vi "GSP_Monitor_handler.vi"(4 "Mode":u16(ring) items=["External", "Internal"], 5 "error in (no error)":errorcluster, 6 "Action":T1, 7 "Motor#":u8, 8 "Monitor Name":string) -> (0 "error out":errorcluster, 2 "Motor# dup":u8)   [LabVIEW 2015]
doc: "Provides an interface for launching and shutting down Silvermax motor monitors. See the action descriptions below:\n\nLaunch - Supply inputs for monitor name (something descriptive), motor#, and mode (encoder type)\n\nShutdown - Shutdown the motor monitor supplied by Motor#\n\nShutdown All - Shutdown all running motor monitors\n\nShow - Open the front panel of the motor monitor supplied by Motor#\n\nHide - Close the front panel of the motor monitor supplied by Motor#"
uses:
  handler_actions.ctl
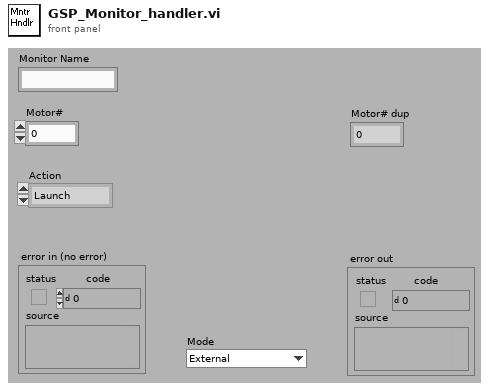
[diagram p1: front panel]
types:
  T1 = typedef "handler_actions.ctl" = enum16{"Launch", "Shutdown All", "Shutdown"}
  T2 = cluster{"Control Name":string, "type string":i16[], "data string":string}
  T3 = cluster{string, "type string":i16[], "data string":string}
  T4 = cluster{"Control Name":string, "type string":i16[], "data string":string}[]
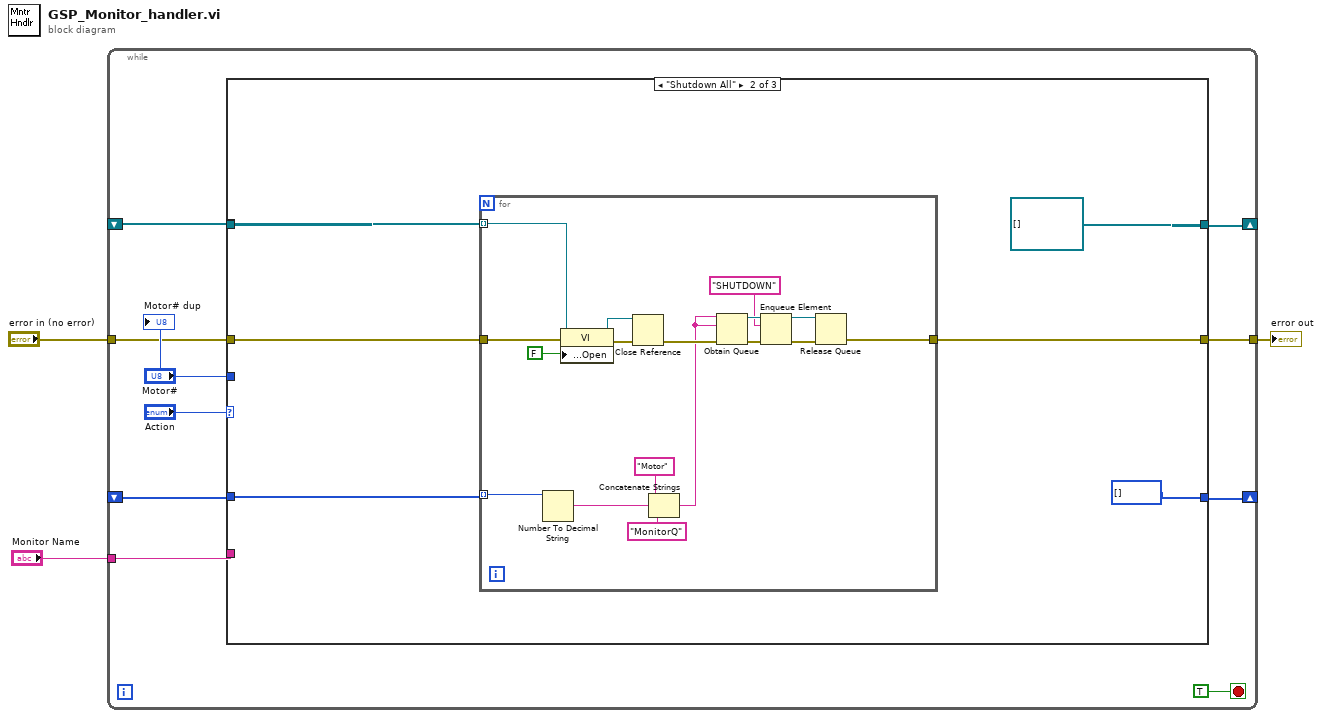
[diagram p0: block diagram]
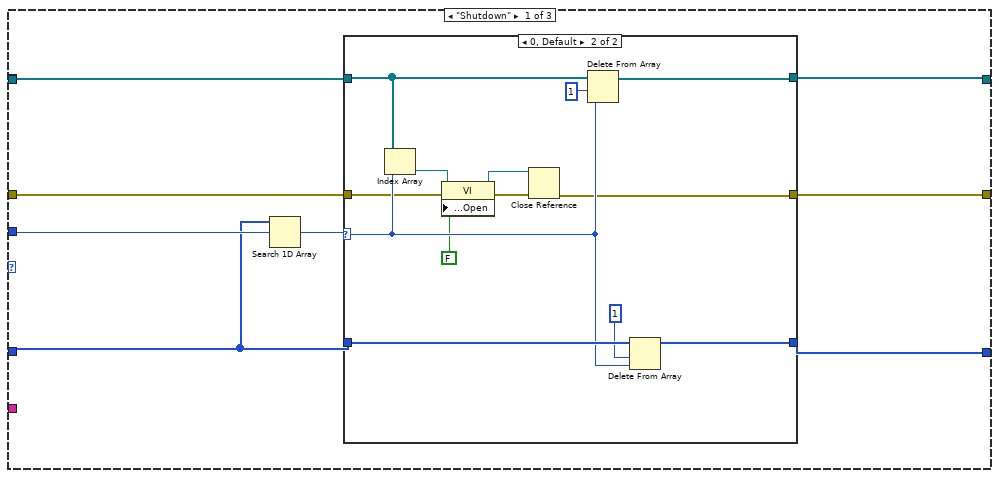
[diagram p2: hidden frame]
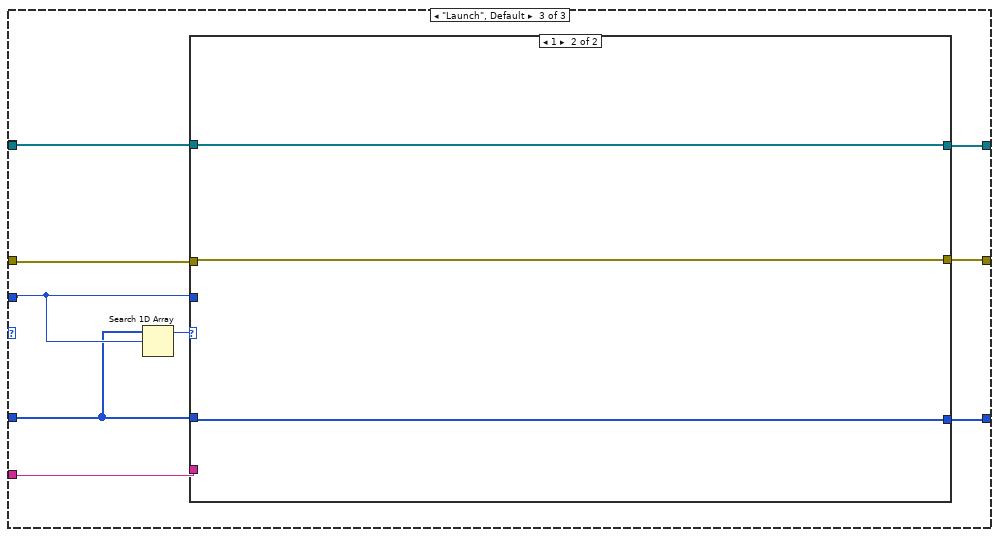
[diagram p4: hidden frame]
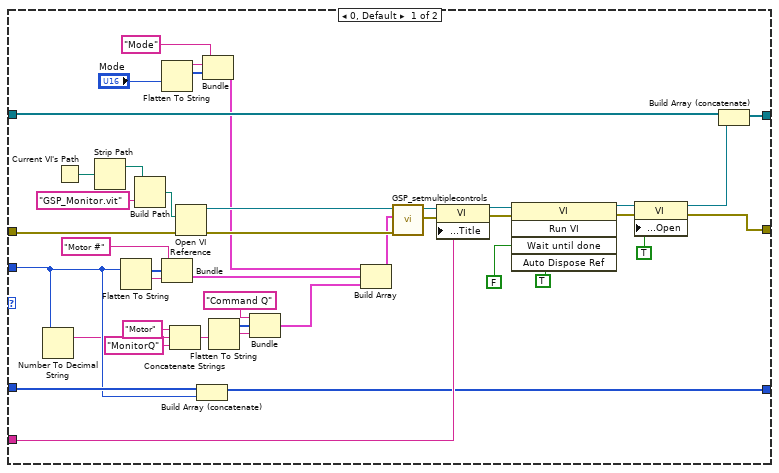
[diagram p5: hidden frame]
diagram:
  n1 = while {
    tunnel: [w13] -> w3
    tunnel: "Monitor Name" -> [w12]
    tunnel: "error in (no error)" -> [w5]
    shift-right: [w9] -> _
    shift-left: _ -> [w4]
    shift-right: [w8] -> _
    shift-left: _ -> [w7]
    stop <- TRUE stop-if-true
    n2 = case shown="\"Shutdown All\"" "Action" {
      tunnel: [w20 w39 w64] -> w13
      tunnel: w12 -> [_ _ w69]
      tunnel: w4 -> [w19 w43 w66]
      tunnel: [w15 refnum<vi>[] [] w67] -> w9
      tunnel: [w14 u8[] [] w65] -> w8
      tunnel: w7 -> [w16 w42 w61]
      tunnel: "Motor#" -> [w18 _ w62]
      tunnel: w5 -> [w21 w40 w68]
      tunnel: w4 -> [_ _ _]
      frame "Shutdown" {
        n3 = Search 1D Array(1D array=w16, element=w18) -> (index of element=w17:i32)  [unwired: 1 in]
        n4 = case shown="0, Default" w17 {
          selector: w17 -> [_ w34]
          tunnel: w21 -> [w24 w31]
          tunnel: [w24 w27] -> w20
          tunnel: w19 -> [w23 w37]
          tunnel: w16 -> [w22 w35]
          tunnel: [w23 w36] -> w15
          tunnel: [w22 w25] -> w14
          frame -1 {
          }
          frame 0, Default {
            n5 = Index Array(array=w37, index=w34) -> (element=w30:refnum<vi>)
            n6 = property class="VI"(reference=w30, error in=w31, "Front Panel Window:Open"=FALSE) -> (reference out=w28:refnum<vi>, error out=w29:errorcluster)
            n7 = Close Reference(reference=w28, error in (no error)=w29) -> (error out=w27:errorcluster)
            n8 = Delete From Array(array=w37, length=1, index=w34) -> (array with subset deleted=w36:refnum<vi>[])  [unwired: 1 out]
            n9 = Delete From Array(array=w35, length=1, index=w34) -> (array with subset deleted=w25:u8[])  [unwired: 1 out]
          }
        }
      }
      frame "Shutdown All" {
        n10 = for {
          tunnel: w42 -> [w53] mode=indexing
          tunnel: w40 -> [w52]
          tunnel: [w49] -> w39
          tunnel: w43 -> [w48] mode=indexing
          n11 = Number To Decimal String(number=w53) -> (decimal integer string=w57:string)  [unwired: 1 in]
          n12 = property class="VI"(reference=w48, error in=w52, "Front Panel Window:Open"=FALSE) -> (reference out=w45:refnum<vi>, error out=w47:errorcluster)
          n13 = Close Reference(reference=w45, error in (no error)=w47) -> (error out=w46:errorcluster)
          n14 = Concatenate Strings("Motor" ("string"), w57, "MonitorQ" ("string")) -> (w44:string)
          n15 = Obtain Queue(name (unnamed)=w44, element data type=w44, error in (no error)=w46) -> (queue out=w56:refnum<queue>, error out=w55:errorcluster)  [unwired: 2 in, 1 out]
          n16 = Enqueue Element(queue=w56, element="SHUTDOWN", error in (no error)=w55) -> (queue out=w51:refnum<queue>, error out=w50:errorcluster)  [unwired: 1 in, 1 out]
          n17 = Release Queue(queue=w51, error in (no error)=w50) -> (error out=w49:errorcluster)  [unwired: 1 in, 2 out]
        }
      }
      frame "Launch", Default {
        n18 = Search 1D Array(1D array=w61, element=w62) -> (index of element=w63:i32)  [unwired: 1 in]
        n19 = case shown="1" w63 {
          tunnel: w69 -> [w105 _]
          tunnel: w68 -> [w104 w113]
          tunnel: [w101 w114] -> w67
          tunnel: w66 -> [w100 w114]
          tunnel: [w99 w112] -> w65
          tunnel: w61 -> [w98 w112]
          tunnel: [w70 w113] -> w64
          tunnel: w62 -> [w97 _]
          frame 0, Default {
            n20 = Number To Decimal String(number=w97) -> (decimal integer string=w95:string)  [unwired: 1 in]
            n21 = Current VI's Path() -> (path=w111:path)
            n22 = Strip Path(path=w111) -> (stripped path=w110:path)  [unwired: 1 out]
            n23 = Flatten To String(anything=w97) -> (data string=w89:string, type string=w90:i16[])  [unwired: 3 in, 1 out]
            n24 = Build Path(base path=w110, name or relative path="GSP_Monitor.vit") -> (appended path=w108:path)
            n25 = Flatten To String(anything="Mode") -> (data string=w78:string, type string=w79:i16[])  [unwired: 3 in, 1 out]
            n26 = Bundle("Control Name"="Motor #", "type string"=w90, "data string"=w89) -> (w85:T2)  [unwired: 1 in]
            n27 = Concatenate Strings("Motor" ("string"), w95, "MonitorQ" ("string")) -> (w93:string)
            n28 = Open VI Reference(vi path=w108, error in (no error)=w104) -> (vi reference=w84:refnum<vi>, error out=w83:errorcluster)  [unwired: 4 in]
            n29 = Build Array (concatenate)(w98, w97) -> (w99:u8[])
            n30 = Bundle("Mode", "type string"=w79, "data string"=w78) -> (w77:T3)  [unwired: 1 in]
            n31 = Flatten To String(anything=w93) -> (data string=w91:string, type string=w92:i16[])  [unwired: 3 in, 1 out]
            n32 = Bundle("Control Name"="Command Q", "type string"=w92, "data string"=w91) -> (w86:T2)  [unwired: 1 in]
            n33 = Build Array(w77, w85, w86) -> (w81:T4)
            n34 = call "GSP_setmultiplecontrols.vi"("error in (no error)"=w83, "Control Infos"=w81, "reference"=w84) -> ("error out"=w82:errorcluster, "reference out"=w80:refnum<vi>)  [unwired: 3 in]
            n35 = property class="VI"(reference=w80, error in=w82, "Front Panel Window:Title"=w105) -> (reference out=w103:refnum<vi>, error out=w102:errorcluster)
            n36 = invoke class="VI" method="Run VI"(reference=w103, error in=w102, "Wait until done"=FALSE, "Auto Dispose Ref"=TRUE) -> (reference out=w74:refnum<vi>, error out=w72:errorcluster)  [unwired: 1 in, 3 out]
            n37 = property class="VI"(reference=w74, error in=w72, "Front Panel Window:Open"=TRUE) -> (reference out=w73:refnum<vi>, error out=w70:errorcluster)
            n38 = Build Array (concatenate)(w100, w73) -> (w101:refnum<vi>[])
          }
          frame 1 {
          }
        }
      }
    }
    "Motor# dup" <- "Motor#"
  }
  "error out" <- w3
